vi "read_attributes.vi"(8 "error in (no error)":errorcluster caption="entrée d'erreur (pas d'erreur)", 11 "Isomap en entrée":refnum<class "Isomap.lvclass">) -> (0 "error out":errorcluster caption="sortie d'erreur", 2 "attributes":T1, 3 "Isomap en sortie":refnum<class "Isomap.lvclass">)   [LabVIEW 2020, in "Isomap.lvclass"]
uses:
  Isomap.lvclass
  Controls/isomap_attributes.ctl
  Isomap.lvclass/Isomap.ctl
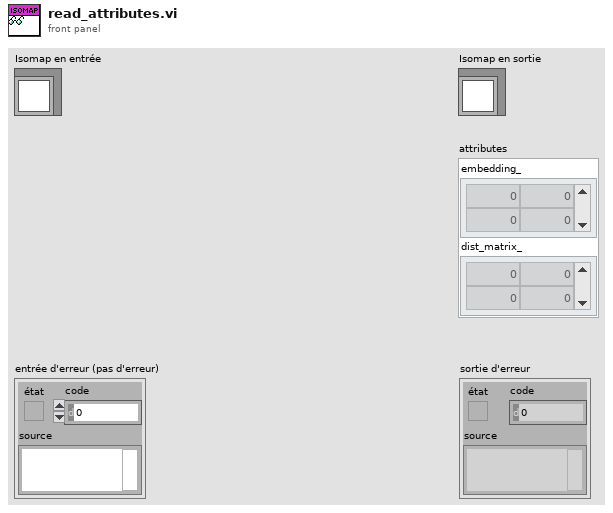
[diagram p1: front panel]
types:
  T1 = typedef "isomap_attributes.ctl" = cluster{"embedding_":dbl[][], "dist_matrix_":dbl[][]}
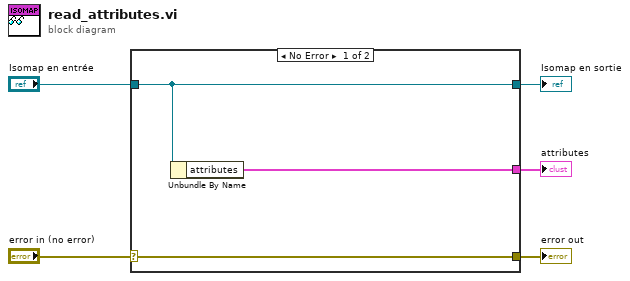
[diagram p0: block diagram]
diagram:
  n1 = case shown="No Error" "error in (no error)" {
    selector: "error in (no error)" -> [w8 w9]
    tunnel: [w8 w9] -> w4
    tunnel: [w7 w10] -> w2
    tunnel: "Isomap en entrée" -> [w7 w10]
    tunnel: [w6 _] -> w1
    frame No Error {
      n2 = Unbundle By Name(w7) -> ("attributes"=w6:T1)
    }
    frame Error {
    }
  }
  "error out" <- w4
  "Isomap en sortie" <- w2
  "attributes" <- w1
